vi "Load_Screen_Ctls.vi"(8 "error out":errorcluster, 10 "CtlRef":refnum<vi>, 11 "Cluster to change":refnum<vi>) -> (0 "error out":errorcluster, 3 "Cluster ref out":refnum<vi>)   [LabVIEW 2020, in "UI_Actor.lvlib" / "UI_Actor.lvclass"]
uses:
  UI_Actor.lvclass
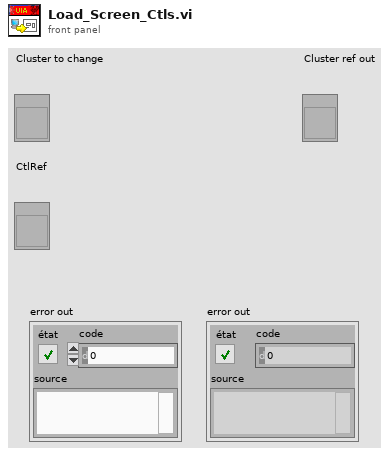
[diagram p1: front panel]
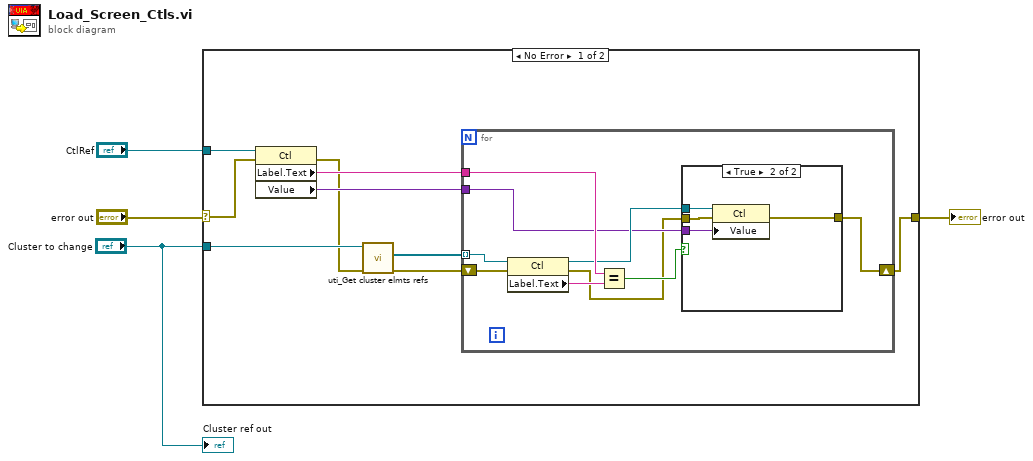
[diagram p0: block diagram]
diagram:
  n1 = case shown="No Error" "error out" {
    selector: "error out" -> [w9 w28]
    tunnel: "CtlRef" -> [w11 _]
    tunnel: [w10 w28] -> w4
    tunnel: "Cluster to change" -> [w8 _]
    frame No Error {
      n2 = property class="Ctl"(reference=w11, error in=w9) -> (error out=w7:errorcluster, "Label.Text"=w12:string, "Value"=w13:variant)  [unwired: 1 out]
      n3 = call "uti_Get cluster elmts refs.vi"("entrée d'erreur (pas d'erreur)"=w7, "Cluster ref in"=w8) -> ("error out"=w5:errorcluster, "Controls[]"=w6:refnum<vi>[])  [unwired: 7 in, 1 out]
      n4 = for {
        tunnel: w12 -> [w21]
        tunnel: w13 -> [w18]
        shift-right: [w17] -> w10
        shift-left: w5 -> [w16]
        tunnel: w6 -> [w14] mode=indexing
        n5 = property class="Ctl"(reference=w14, error in=w16) -> (reference out=w19:refnum<vi>, error out=w15:errorcluster, "Label.Text"=w22:string)
        n6 = Equal?(x=w21, y=w22) -> (x = y?=w20:bool)
        n7 = case shown="True" w20 {
          tunnel: w19 -> [_ w27]
          tunnel: w18 -> [_ w26]
          tunnel: [w23 w25] -> w17
          tunnel: w15 -> [w23 w24]
          frame False {
          }
          frame True {
            n8 = property class="Ctl"(reference=w27, error in=w24, "Value"=w26) -> (error out=w25:errorcluster)  [unwired: 1 out]
          }
        }
      }
    }
    frame Error {
    }
  }
  "error out" <- w4
  "Cluster ref out" <- "Cluster to change"
